vi "Emballage_BDD_choix_Config_imprimante.vi"(8 "Error in":errorcluster caption="Error in (no error)") -> (0 "Error out":errorcluster, 1 "imprimante Certificats 2":string(combo), 2 "Dec. Droite":string="^LH70,20", 3 "imprimante Etiquettes OUT":string, 4 "Indice Imprimante":i32, 5 "Liste IP":string[](array[string]))   [LabVIEW 2020]
uses:
  Modules/FS/60_FS_Controles/60_FS_SetGet.ctl
  <vilib>/Utility/NIReport.llb/NI_ReportGenerationCore.lvlib
panel:
  in  "imprimante Certificats":string(combo)
  in  "Dec. Droite 2":string="^LH70,20"
  in  "imprimante Etiquettes":string(combo)
  in  "Bouton OK":bool
  # "Veuillez sélectionner les imprimantes!!"
  # "Vous pouvez changer le décalage à droite:"
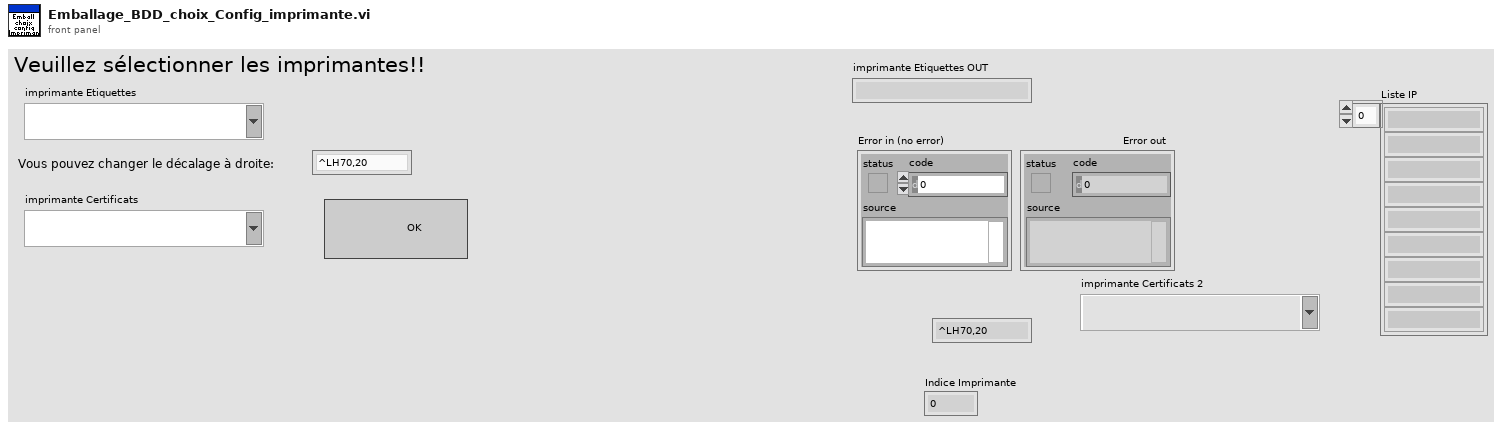
[diagram p1: front panel]
types:
  T1 = typedef "60_FS_SetGet.ctl" = enum16{"set", "get"}
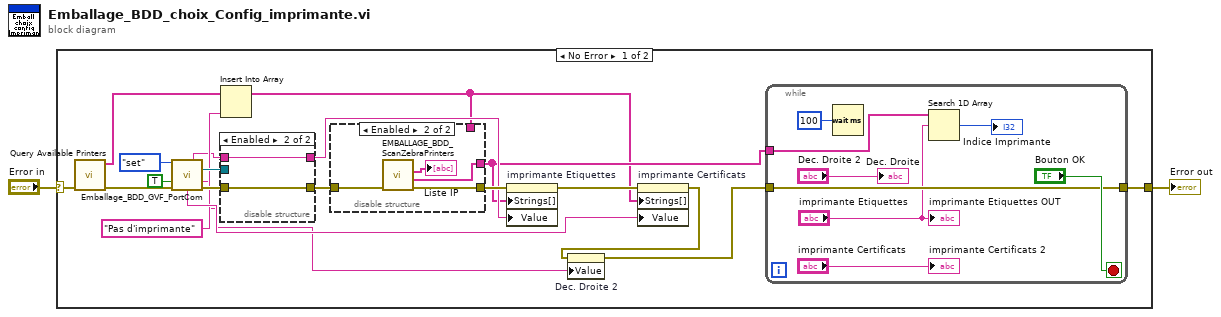
[diagram p0: block diagram]
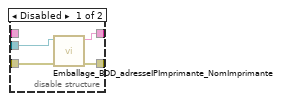
[diagram p2: hidden frame]
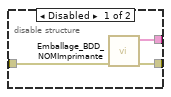
[diagram p3: hidden frame]
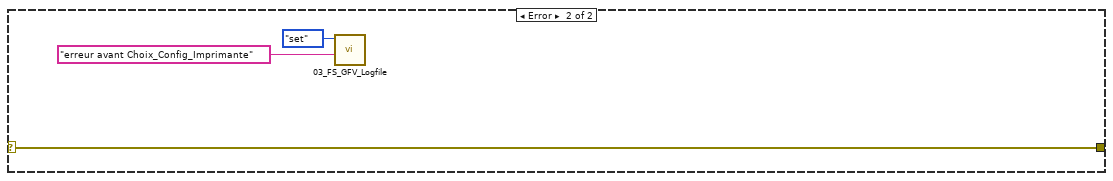
[diagram p4: hidden frame]
diagram:
  n1 = case shown="No Error" "Error in" {
    selector: "Error in" -> [w15 w46]
    tunnel: [w17 w46] -> w1
    frame No Error {
      n2 = call <vilib>:"Query Available Printers.vi"("error in (no error)"=w15) -> ("error out"=w14:errorcluster, "system configured printers"=w11:string[])  [unwired: 8 in, 1 out]
      n3 = call "Emballage_BDD_GVF_PortCom.vi"("Énum"=enum16{"get", "set"}."set", "bdd"=TRUE, "Error in"=w14) -> ("Imprimante Zebra"=w10:string, "PortCom imprimante OUT"=w18:refnum<visa-resource-name>, "DecDroit_OUT"=w7:string, "Imprimante Certif."=w13:string, "Error out"=w20:errorcluster)  [unwired: 6 in, 2 out]
      n4 = Insert Into Array(array=w11, new element="Pas d'imprimante" ("nouvel élément/sous-tableau")) -> (w3:string[])  [unwired: 1 in]
      n5 = disable-structure shown="Enabled" {
        disable-tunnel: w20 -> [w26 w28]
        disable-tunnel: [w25 w27] -> w5
        disable-tunnel: [w24 w28] -> w19
        disable-tunnel: w18 -> [w23 _]
        disable-tunnel: w10 -> [_ w27]
        frame Disabled {
          n6 = call "Emballage_BDD_adresseIPImprimante_NomImprimante.vi"("Error in"=w26, "ADRESSE_IP"=w23) -> ("Error out"=w24:errorcluster, "NOM"=w25:string)  [unwired: 8 in]
        }
        frame Enabled {
        }
      }
      n7 = disable-structure shown="Enabled" {
        disable-tunnel: [w31 w34] -> w22
        disable-tunnel: [w30 w35] -> w4
        disable-tunnel: w19 -> [w29 w33]
        disable-tunnel: w3 -> [_ _]
        frame Disabled {
          n8 = call "Emballage_BDD_NOMImprimante.vi"("Error in"=w29) -> ("Error out"=w31:errorcluster, "élément"=w30:string[])  [unwired: 9 in]
        }
        frame Enabled {
          n9 = call "EMBALLAGE_BDD_ScanZebraPrinters.vi"("error in (no error)"=w33) -> ("error out"=w34:errorcluster, "Liste Nom"=w35:string[], "Liste IP"=→"Liste IP":string[])  [unwired: 7 in, 1 out]
        }
      }
      n10 = property on="imprimante Etiquettes" class="CmbBox"(error in=w22, "Strings[]"=w4, "Value"=w5) -> (error out=w16:errorcluster)  [unwired: 1 in, 1 out]
      n11 = property on="imprimante Certificats" class="CmbBox"(error in=w16, "Strings[]"=w3, "Value"=w13) -> (error out=w9:errorcluster)  [unwired: 1 in, 1 out]
      n12 = property on="Dec. Droite 2" class="Str"(error in=w9, "Value"=w7) -> (error out=w8:errorcluster)  [unwired: 1 in, 1 out]
      n13 = while {
        tunnel: [w42] -> w17
        tunnel: w8 -> [w42]
        tunnel: w4 -> [w37]
        stop <- "Bouton OK" stop-if-true
        n14 = Wait (ms)(milliseconds to wait=u32 100 ("attente (ms)")) -> ()  [unwired: 1 out]
        n15 = Search 1D Array(1D array=w37, element="imprimante Etiquettes") -> (index of element=→"Indice Imprimante":i32)  [unwired: 1 in]
        "imprimante Etiquettes OUT" <- "imprimante Etiquettes"
        "Dec. Droite" <- "Dec. Droite 2"
        "imprimante Certificats 2" <- "imprimante Certificats"
      }
    }
    frame Error {
      n16 = call "03_FS_GFV_Logfile.vi"("Chaîne"="erreur avant Choix_Config_Imprimante", "States"=60_FS_SetGet."set") -> ()  [unwired: 8 in, 2 out]
    }
  }
  "Error out" <- w1
